vi "configuration UI.vi"() -> ()   [LabVIEW 2013, in "Modbus Slave editor node.lvclass"]
doc: "Platypus Framework 1.0.1.65\nNI Systems Engineering - National Instruments"
uses:
  Modbus Slave editor node.lvclass
  <vilib>/NI/Configuration Framework/Node/NodeRef.ctl
  <vilib>/NI/Configuration Framework/Node/NISE_CEF_Node.lvclass
  <vilib>/NI/AMC/Message Queue.ctl
  <vilib>/NI/AMC/Message.ctl
  <vilib>/NI/Tools/Keyed Array/KeyedArray.ctl
  <vilib>/NI/Configuration Framework/Node/UserEventRef.ctl
  <vilib>/NI/Configuration Framework/Controls/EventCluster.ctl
  module/configuration/modbus mapping behavior.ctl
  module/configuration/modbus class.ctl
  <vilib>/NI/Module Execution Interface/Engine Configuration/engine configuration.lvclass
  module/configuration/Modbus Slave configuration.lvclass
  <vilib>/NI/Tag Bus Data Framework/Configuration Editor/Classes/Engine Parent/Engine Parent Editor Node.lvclass
  <vilib>/NI/Tag Bus/tag/tag descriptor.lvclass
  <vilib>/NI/Tag Bus/tag/Data Type.ctl
  <vilib>/NI/Tag Bus/tag/tag descriptor.lvclass/tag descriptor.ctl
  <vilib>/NI/Configuration Framework/serializable configuration/NISE_CEF_serializable configuration.lvclass/NISE_CEF_serializable configuration.ctl
  <vilib>/NI/Configuration Framework/serializable configuration/NISE_CEF_serializable configuration.lvclass
  module/configuration/Modbus Slave configuration.lvclass/Modbus Slave configuration.ctl
  Modbus Slave editor node.lvclass/Modbus Slave editor node.ctl
  <vilib>/NI/Tag Bus/tag/write data type.vi
  module/configuration/Write port (502).vi
  module/configuration/Write baud rate.vi
  module/configuration/Write class.vi
  module/configuration/Write flow control (none).vi
  module/configuration/Write parity (even).vi
  module/configuration/Write serial type.vi
  module/configuration/Write unit ID.vi
  module/configuration/Write VISA resource name.vi
  module/configuration/Write IP address.vi
  module/configuration/Read modbus channels.vi
  module/configuration/Read port (502).vi
  module/configuration/Read baud rate.vi
  module/configuration/Read class.vi
  module/configuration/Read flow control (none).vi
  module/configuration/Read parity (even).vi
  module/configuration/Read serial type.vi
  module/configuration/Read unit ID.vi
  module/configuration/Read VISA resource name.vi
  module/configuration/Read IP address.vi
  <vilib>/NI/Tag Bus Data Framework/Configuration Editor/Classes/Module editor node/Read Module Configuration.vi
  <vilib>/NI/Tag Bus Module Framework/module configuration/TBM module configuration.lvclass
  module/module channel/Modbus Module Channel.lvclass
  <vilib>/NI/Configuration Framework/NISE_CEF_TreeControl.lvlib
  <vilib>/NI/Tag Bus Data Framework/Configuration Editor/Classes/Module editor node/module editor node.lvclass
  <vilib>/NI/Tools/Keyed Array/Tools_KeyedArray.lvlib
  <vilib>/NI/AMC/AMC.lvlib
panel:
  in  "export":bool
  in  "Tab Control":T1(tab)
  in  "hidden_remove":bool
  in  "hidden_settings":bool
  in  "hidden_Add":bool
  in  "Remove Button":bool
  in  "Add Button":bool
  in  "channel":i32(listbox)=1
  in  "settings":bool
  in  "address":string
  in  "port (502)":u16=502
  in  "baud rate":u32
  in  "class":T2
  in  "flow control (none)":u16
  in  "parity (even)":u16
  in  "serial type":enum16{"RTU", "ASCII"}(ring)
  in  "unit ID":u8
  in  "VISA resource name":refnum<visa-resource-name>
  in  "remap":bool
  in  "mapping":T3
  in  "user event":T4
  in  "main queue":T5
  in  "node ref":T6
  # "TCP"
  # "TCP Master"
  # "Serial"
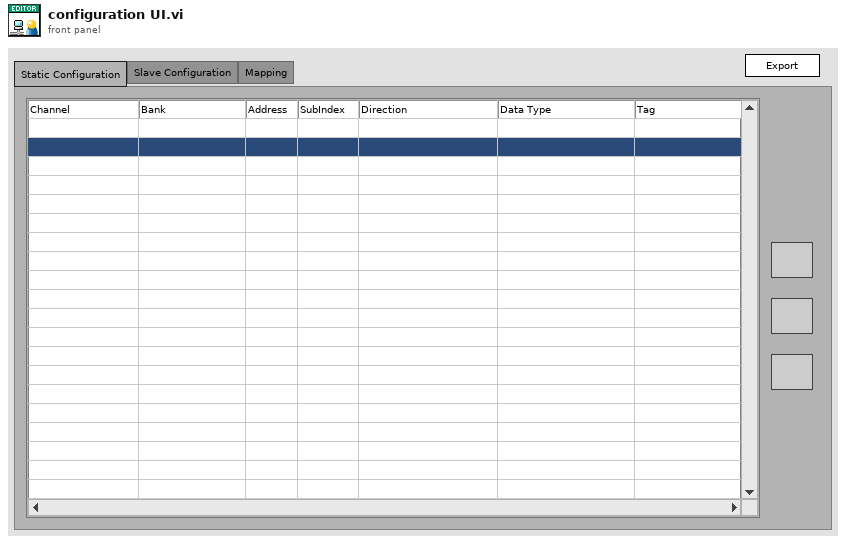
[diagram p1: front panel]
types:
  T1 = enum32{"Static Configuration", "Slave Configuration", "Mapping"}
  T2 = typedef "Modbus Slave configuration.lvclass/modbus class.ctl" = enum16{"TCP master", "TCP slave", "serial master", "serial slave"}
  T3 = typedef "Modbus Slave configuration.lvclass/modbus mapping behavior.ctl" = enum16{"custom", "optimized"}
  T4 = typedef "NISE_CEF_Node.lvclass/UserEventRef.ctl" = refnum<user-event>
  T5 = typedef "AMC.lvlib/Message Queue.ctl" = refnum<queue>
  T6 = typedef "NISE_CEF_Node.lvclass/NodeRef.ctl" = refnum<data-value>
  T7 = typedef "NISE_CEF_TreeControl.lvlib/EventCluster.ctl" = cluster{"command":string, "data":string}
  T8 = typedef "tag bus.lvlib/tag descriptor.lvclass/Data Type.ctl" = enum16{"Double", "Single", "I64", "I32", "I16", "I8", "U64", "U32", "U16", "U8", "Boolean", "String", "Array of Double", "Array of Single", "Array of I64", "Array of I32", "Array of I16", "Array of I8", "Array of U64", "Array of U32", "Array of U16", "Array of U8", "Array of Boolean", "Array of String"}
  T9 = typedef "Modbus Slave editor node.lvclass/table line.ctl" = cluster{"mbchan":refnum<class "Modbus Module Channel.lvclass">, "tag name":string}
  T10 = typedef "LVPoint32TypeDef.ctl" = cluster{"Horizontal":i32, "Vertical":i32}
  T11 = typedef "LVRowAndColumnTypeDef.ctl" = cluster{"Row":i32, "Column":i32}
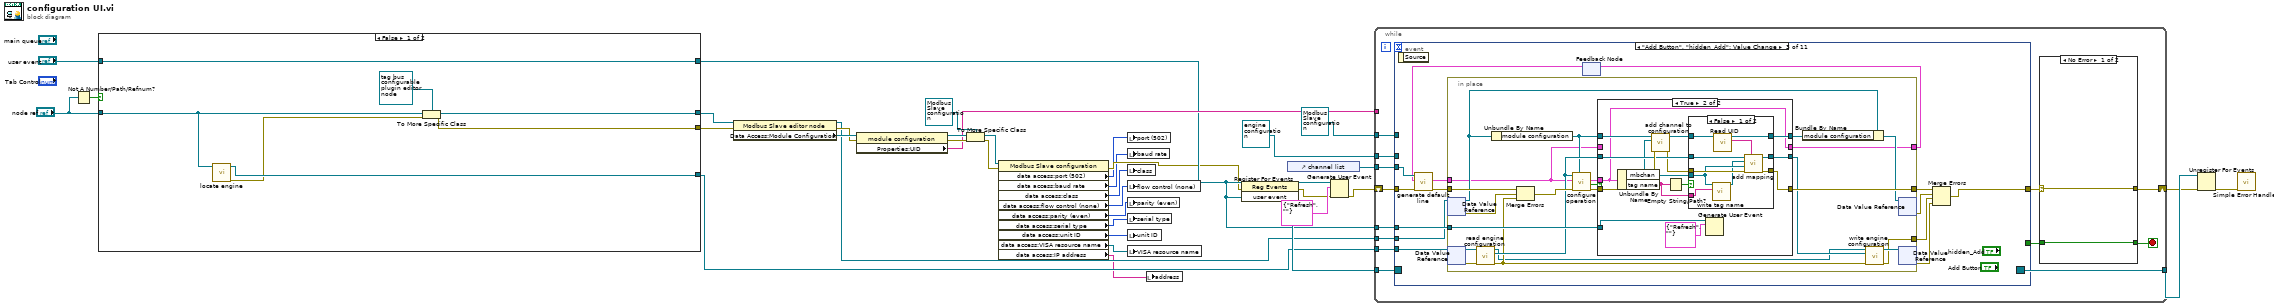
[diagram p0: block diagram]
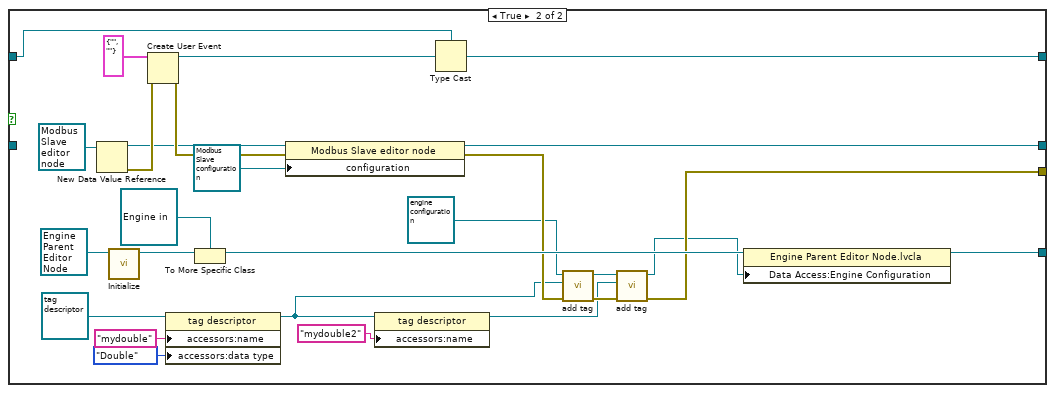
[diagram p2: hidden frame]
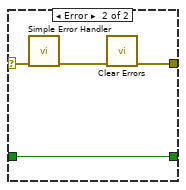
[diagram p3: hidden frame]
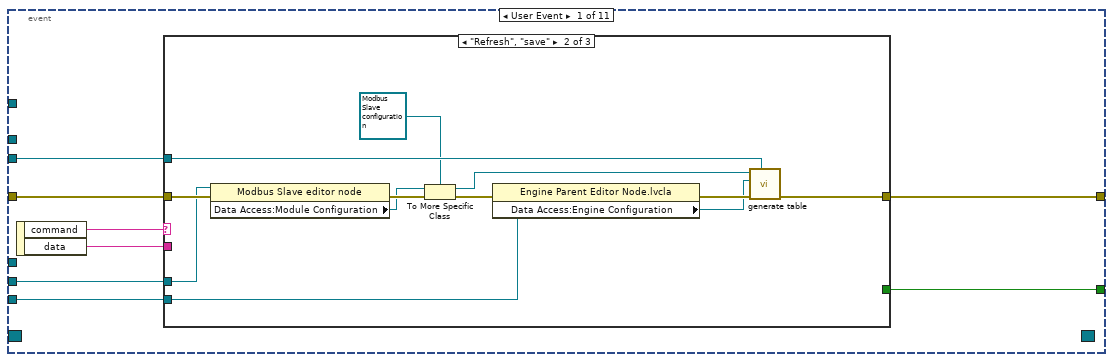
[diagram p4: hidden frame]
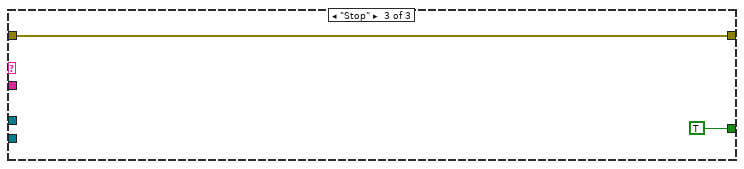
[diagram p6: hidden frame]
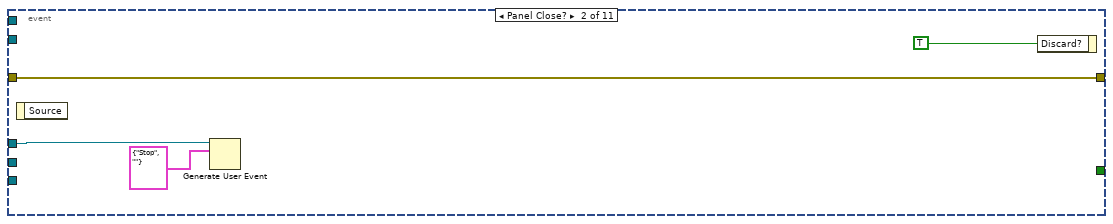
[diagram p7: hidden frame]
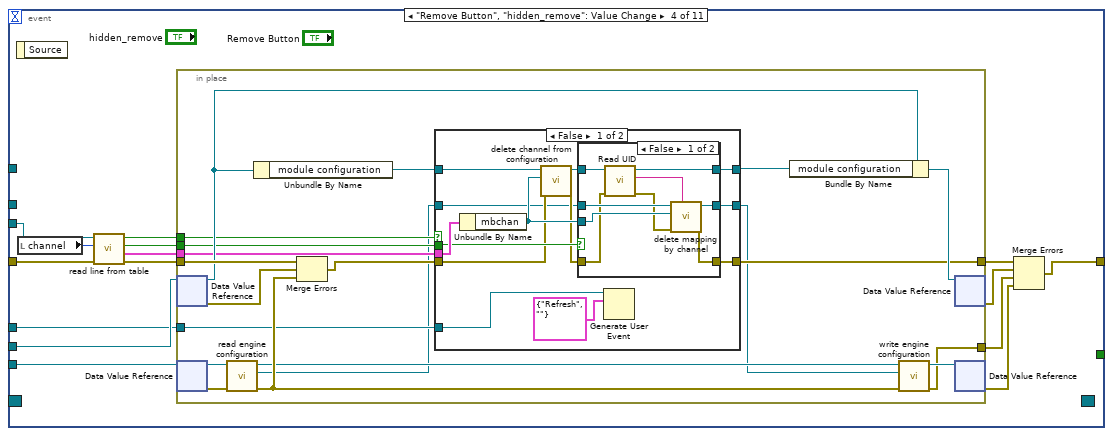
[diagram p10: hidden frame]
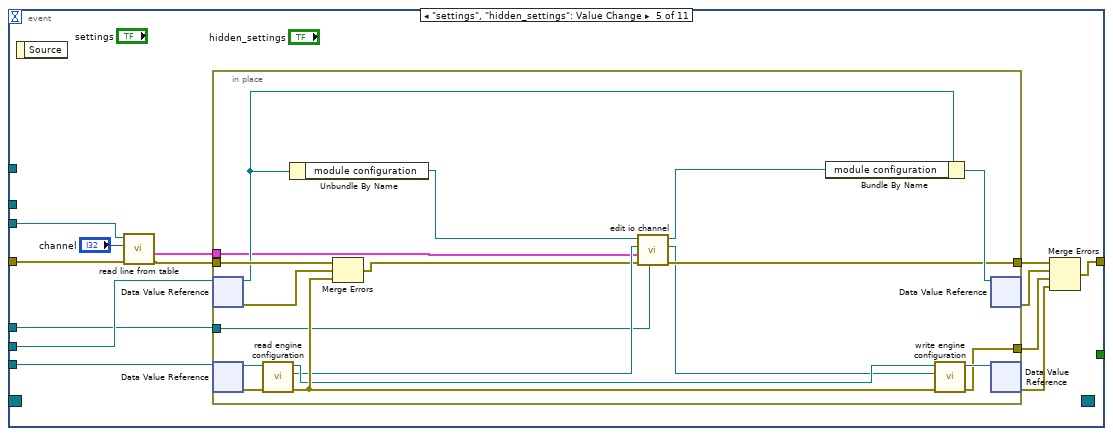
[diagram p13: hidden frame]
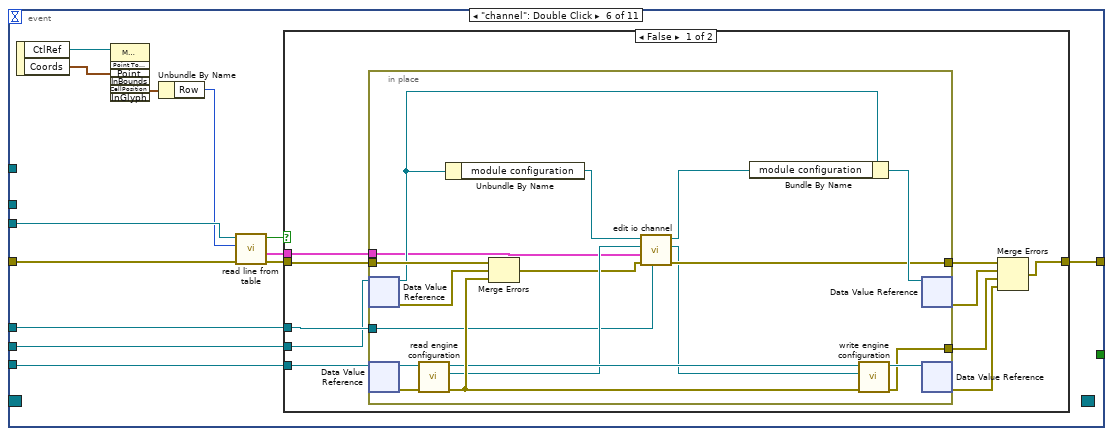
[diagram p14: hidden frame]
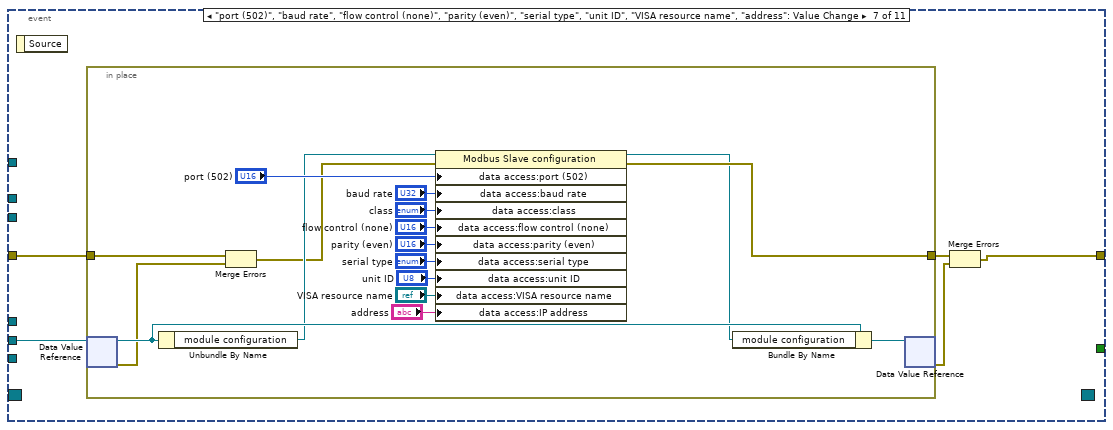
[diagram p16: hidden frame]
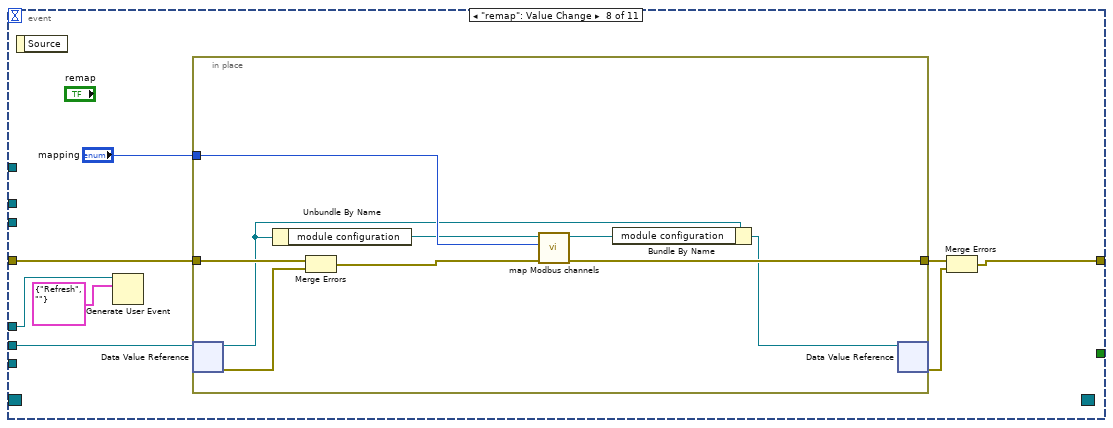
[diagram p17: hidden frame]
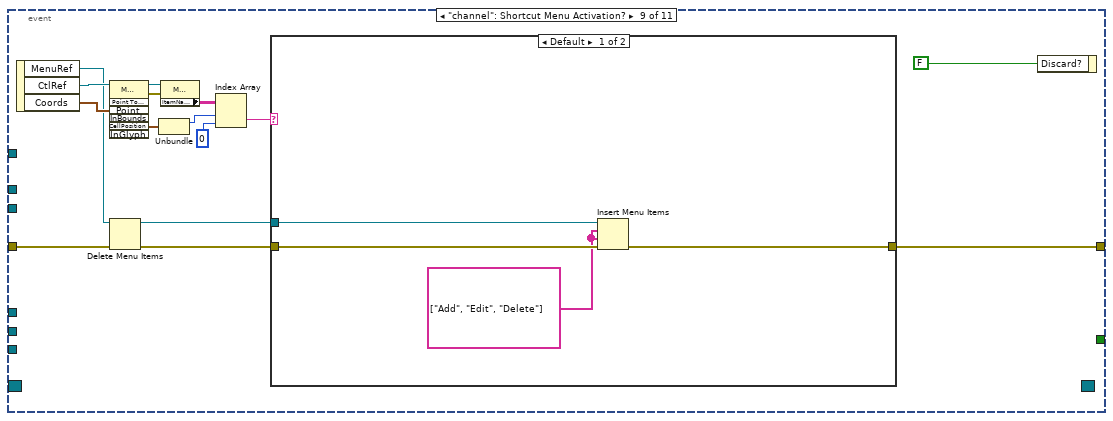
[diagram p18: hidden frame]
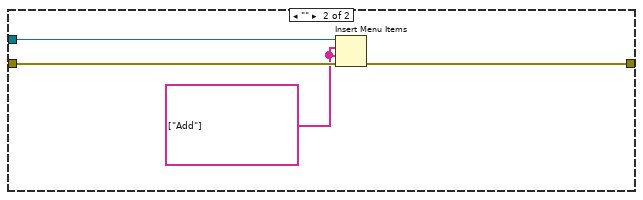
[diagram p19: hidden frame]
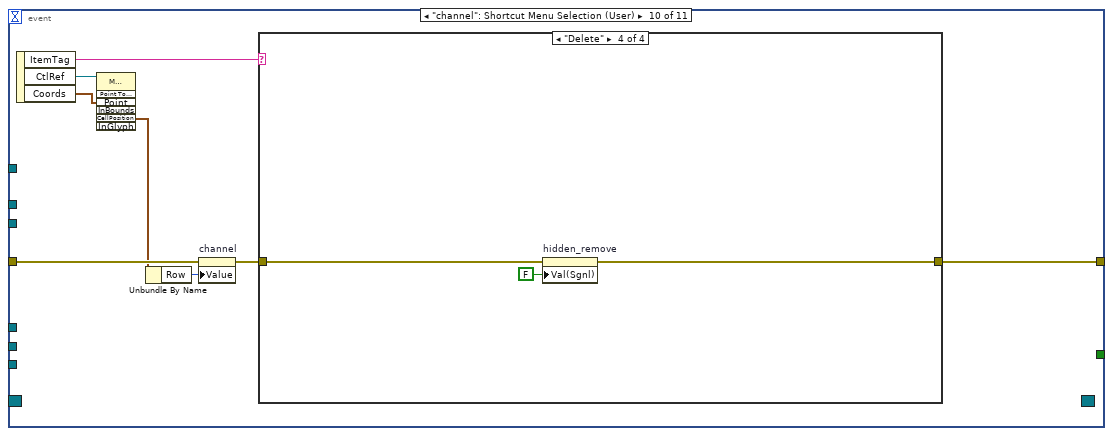
[diagram p20: hidden frame]
diagram:
  n1 = Not A Number/Path/Refnum?(number/path/refnum="node ref") -> (NaN/Path/Refnum?=w28:bool)
  n2 = case shown="False" w28 {
    tunnel: "user event" -> [w43 w47]
    tunnel: [w43 w48] -> w15
    tunnel: "node ref" -> [w41 _]
    tunnel: [w40 w64] -> w23
    tunnel: [w39 w51] -> w26
    tunnel: [w38 w45] -> w21
    frame False {
      n3 = call <vilib>:"locate engine.vi"("component"=w41) -> ("error out"=w37:errorcluster, "engine"=w38:refnum<data-value>)  [unwired: 9 in]
      n4 = To More Specific Class(target class=refnum<data-value> refnum ("data value reference"), reference=w41, error in=w37) -> (specific class reference=w40:refnum<data-value>, error out=w39:errorcluster)
    }
    frame True {
      n5 = New Data Value Reference(data value=refnum<class "Modbus Slave editor node.lvclass"> refnum ("tag bus configurable plugin editor node")) -> (data value reference=w63:refnum<data-value>, error out=w66:errorcluster)  [unwired: 1 in]
      n6 = call-dynamic "Initialize.vi"("Engine in"=refnum<class "Engine Parent Editor Node.lvclass"> refnum) -> ("data value reference"=w62:T6)  [unwired: 8 in, 2 out]
      n7 = Create User Event(user event datatype=T7 {"command"="", "data"=""} ("event data"), error in=w66) -> (user event=w69:refnum<user-event>, error out=w65:errorcluster)
      n8 = property class="tag descriptor"(reference=refnum<class "tag descriptor.lvclass"> refnum ("tag descriptor"), "accessors:name"="mydouble" ("name"), "accessors:data type"=Data_Type."Double" ("data type")) -> (reference out=w49:refnum<class "tag descriptor.lvclass">)  [unwired: 1 in, 1 out]
      n9 = To More Specific Class(target class=refnum<data-value> refnum ("data value reference"), reference=w62) -> (specific class reference=w61:refnum<data-value>)  [unwired: 1 in, 1 out]
      n10 = property class="Modbus Slave editor node"(reference=w63, error in=w65, "configuration"=refnum<class "Modbus Slave configuration.lvclass"> refnum ("tag bus configurable plugin module configuration")) -> (reference out=w64:refnum<data-value>, error out=w55:errorcluster)
      n11 = property class="tag descriptor"(reference=w49, "accessors:name"="mydouble2" ("name")) -> (reference out=w50:refnum<class "tag descriptor.lvclass">)  [unwired: 1 in, 1 out]
      n12 = Type Cast(type=w47, x=w69) -> (*(type *) &x=w48:T4)
      n13 = call <vilib>:"add tag.vi"("error in"=w55, "tag descriptor"=w49, "engine configuration in"=refnum<class "engine configuration.lvclass"> refnum ("Engine Configuration")) -> ("error out"=w53:errorcluster, "engine configuration out"=w52:refnum<class "engine configuration.lvclass">)  [unwired: 7 in]
      n14 = call <vilib>:"add tag.vi"("error in"=w53, "tag descriptor"=w50, "engine configuration in"=w52) -> ("error out"=w51:errorcluster, "engine configuration out"=w44:refnum<class "engine configuration.lvclass">)  [unwired: 7 in]
      n15 = property class="Engine Parent Editor Node.lvcla"(reference=w61, "Data Access:Engine Configuration"=w44) -> (reference out=w45:refnum<data-value>)  [unwired: 1 in, 1 out]
    }
  }
  n16 = property class="Modbus Slave editor node"(reference=w23, error in=w26) -> (reference out=w22:refnum<data-value>, error out=w31:errorcluster, "Data Access:Module Configuration"=w32:refnum<class "TBM module configuration.lvclass">)
  n17 = property class="module configuration"(reference=w32, error in=w31) -> (reference out=w29:refnum<class "TBM module configuration.lvclass">, error out=w30:errorcluster, "Properties:UID"=w25:string)
  n18 = To More Specific Class(target class=refnum<class "Modbus Slave configuration.lvclass"> refnum ("tag bus configurable plugin module configuration"), reference=w29, error in=w30) -> (specific class reference=w12:refnum<class "Modbus Slave configuration.lvclass">, error out=w11:errorcluster)
  n19 = property class="Modbus Slave configuration"(reference=w12, error in=w11) -> (error out=w10:errorcluster, "data access:port (502)"=w5:u16, "data access:baud rate"=w9:u32, "data access:class"=w6:T2, "data access:flow control (none)"=w4:u16, "data access:parity (even)"=w3:u16, "data access:serial type"=w2:enum16{"RTU", "ASCII"}, "data access:unit ID"=w7:u8, "data access:VISA resource name"=w8:refnum<visa-resource-name>, "data access:IP address"=w1:string)  [unwired: 1 out]
  n20 = local write "port (502)"(w5) -> ()
  n21 = local write "baud rate"(w9) -> ()
  n22 = local write "class"(w6) -> ()
  n23 = local write "flow control (none)"(w4) -> ()
  n24 = local write "parity (even)"(w3) -> ()
  n25 = local write "serial type"(w2) -> ()
  n26 = local write "unit ID"(w7) -> ()
  n27 = local write "VISA resource name"(w8) -> ()
  n28 = local write "address"(w1) -> ()
  n29 = register-events(error in=w10, w15) -> (reference out=w36:refnum<event-registration>, error out=w14:errorcluster)  [unwired: 1 in]
  n30 = control-ref of="channel list"() -> (w19:refnum<vi>)
  n31 = Generate User Event(user event=w15, event data cluster=T7 {"command"="Refresh", "data"=""} ("event data"), error in=w14) -> (error out=w13:errorcluster)  [unwired: 1 in, 1 out]
  n32 = while {
    tunnel: w36 -> [w83]
    tunnel: [w82] -> w35
    shift-right: [w79] -> w34
    shift-left: w13 -> [w81]
    tunnel: w25 -> [_]
    tunnel: w22 -> [w76]
    tunnel: w21 -> [w75]
    tunnel: w15 -> [w74]
    tunnel: w19 -> [w72]
    tunnel: refnum<class "Modbus Slave configuration.lvclass"> refnum ("tag bus configurable plugin module configuration") -> [w78]
    tunnel: refnum<class "engine configuration.lvclass"> refnum ("Engine Configuration") -> [w77]
    stop <- w80 stop-if-true
    n33 = event shown="[2] \"Add Button\", \"hidden_Add\": Value Change" {
      selector: w83 -> [_ _ _ _ _ _ _ _ _ _ _]
      dyn-events: [_ _ _ _ _ _ _ _ _ _ _] -> w82
      timeout: _ -> [_ _ _ _ _ _ _ _ _ _ _]
      tunnel: [w97 _ _ _ _ _ _ _ _ _ _] -> w71
      tunnel: [w91 w116 w124 w187 w252 w289 w321 w344 w359 w386 w408] -> w73
      tunnel: w81 -> [w92 w116 w129 w198 w259 w290 w324 w349 w373 w385 w413]
      tunnel: w78 -> [_ _ _ _ _ _ _ _ _ _ _]
      tunnel: w77 -> [_ _ _ _ _ _ _ _ _ _ _]
      tunnel: w76 -> [w95 _ w120 w189 w248 w279 w322 w342 _ _ w406]
      tunnel: w75 -> [w94 _ w123 w190 w249 w278 _ _ _ _ _]
      tunnel: w74 -> [_ w113 w126 w188 w247 w286 _ w347 _ _ _]
      tunnel: w72 -> [w90 _ w125 w196 w257 w285 _ _ _ _ _]
      event User Event {
        n34 = event-data() -> ("command"=w96:string, "data"=w93:string)  [unwired: 1 in]
        n35 = case shown="\"Refresh\", \"save\"" w96 {
          tunnel: [_ _ TRUE] -> w97
          tunnel: w95 -> [_ w105 _]
          tunnel: w94 -> [_ w104 _]
          tunnel: w93 -> [_ _ _]
          tunnel: w92 -> [w98 w110 w111]
          tunnel: [w98 w109 w111] -> w91
          tunnel: w90 -> [_ w108 _]
          frame Default {
          }
          frame "Refresh", "save" {
            n36 = property class="Modbus Slave editor node"(reference=w105, error in=w110) -> (error out=w106:errorcluster, "Data Access:Module Configuration"=w100:refnum<class "TBM module configuration.lvclass">)  [unwired: 1 out]
            n37 = To More Specific Class(target class=refnum<class "Modbus Slave configuration.lvclass"> refnum ("tag bus configurable plugin module configuration"), reference=w100, error in=w106) -> (specific class reference=w99:refnum<class "Modbus Slave configuration.lvclass">, error out=w102:errorcluster)
            n38 = property class="Engine Parent Editor Node.lvcla"(reference=w104, error in=w102) -> (error out=w107:errorcluster, "Data Access:Engine Configuration"=w103:refnum<class "engine configuration.lvclass">)  [unwired: 1 out]
            n39 = call "generate table.vi"("table"=w108, "error in"=w107, "engine configuration"=w103, "tag bus configurable plugin module configuration"=w99) -> ("error out"=w109:errorcluster)  [unwired: 7 in]
          }
          frame "Stop" {
          }
        }
      }
      event Panel Close? {
        n40 = event-data() -> ()  [unwired: 1 in, 1 out]
        n41 = Generate User Event(user event=w113, event data cluster=T7 {"command"="Stop", "data"=""} ("event data")) -> ()  [unwired: 2 in, 2 out]
        n42 = event-data("Discard?"=TRUE) -> ()  [unwired: 1 in, 1 out]
      }
      event "Add Button", "hidden_Add": Value Change {
        n43 = event-data() -> ()  [unwired: 1 in, 1 out]
        n44 = feedback #1() -> (w117:T9)  [unwired: 1 in]
        n45 = call "generate default line.vi"("error in"=w129, "last line"=w117, "operations table"=w125) -> ("error out"=w127:errorcluster, "line"=w128:T9)  [unwired: 7 in]
        n46 = in-place {
          in-place-border: [w152] -> w130
          in-place-border: w128 -> [w132]
          in-place-border: w127 -> [w151]
          in-place-border: w126 -> [w147]
          in-place-border: [w138] -> w121
          in-place-border: [w131] -> w118
          n47 = in-place-dvr #2(w120) -> (w133:refnum<class "Modbus Slave editor node.lvclass">, w137:errorcluster)
          n48 = in-place-dvr #3(w123) -> (w145:refnum<class "Engine Parent Editor Node.lvclass">, w144:errorcluster)
          n49 = call <vilib>:"read engine configuration.vi"("error in"=w144, "Engine Parent Editor Node in"=w145) -> ("error out"=w140:errorcluster, "engine configuration"=w143:refnum<class "engine configuration.lvclass">, "Engine Parent Editor Node out"=w139:refnum<class "Engine Parent Editor Node.lvclass">)  [unwired: 7 in]
          n50 = Unbundle By Name(w133) -> ("module configuration"=w136:refnum<class "Modbus Slave configuration.lvclass">)
          n51 = Merge Errors(w151, w137, w140) -> (w146:errorcluster)
          n52 = call "configure operation.vi"("tag bus configurable plugin module configuration"=w136, "error in"=w146, "line item in"=w132, "engine configuration"=w143) -> ("error out"=w149:errorcluster, "success"=w148:bool, "line item out"=w150:T9)  [unwired: 4 in, 1 out]
          n53 = case shown="True" w148 {
            tunnel: [w156 w160] -> w152
            tunnel: w149 -> [w156 w169]
            tunnel: w143 -> [w155 w167]
            tunnel: w150 -> [_ w157]
            tunnel: w136 -> [w154 w170]
            tunnel: [w155 w166] -> w141
            tunnel: [w154 w161] -> w135
            tunnel: w147 -> [_ w159]
            tunnel: w132 -> [w153 _]
            tunnel: [w153 w157] -> w131
            frame False {
            }
            frame True {
              n54 = Unbundle By Name(w157) -> ("mbchan"=w164:refnum<class "Modbus Module Channel.lvclass">, "tag name"=w163:string)
              n55 = call "add channel to configuration.vi"("error in"=w169, "Modbus Module Channel.lvclass"=w164, "Modbus Slave configuration in"=w170) -> ("error out"=w165:errorcluster, "Modbus Slave configuration out"=w162:refnum<class "Modbus Slave configuration.lvclass">)  [unwired: 7 in]
              n56 = Empty String/Path?(string/path=w163) -> (empty?=w168:bool)
              n57 = case shown="False" w168 {
                tunnel: w167 -> [w180 w183]
                tunnel: [w179 w183] -> w166
                tunnel: w165 -> [w178 w182]
                tunnel: w164 -> [w175 _]
                tunnel: w163 -> [w173 _]
                tunnel: [w177 w182] -> w160
                tunnel: w162 -> [w176 w181]
                tunnel: [w172 w181] -> w161
                frame False {
                  n58 = call <vilib>:"write tag name.vi"("name"=w173, "system tag in"=w175) -> ("system tag out"=w174:refnum<class "Modbus Module Channel.lvclass">)  [unwired: 8 in, 1 out]
                  n59 = call <vilib>:"Read UID.vi"("configuration in"=w176) -> ("instance id"=w171:string, "configuration out"=w172:refnum<class "Modbus Slave configuration.lvclass">)  [unwired: 8 in, 1 out]
                  n60 = call <vilib>:"add mapping.vi"("owner ID"=w171, "error in"=w178, "channel"=w175, "tag descriptor"=w174, "engine configuration"=w180) -> ("error out"=w177:errorcluster, "engine configuration out"=w179:refnum<class "engine configuration.lvclass">)  [unwired: 5 in]
                }
                frame True {
                }
              }
              n61 = Generate User Event(user event=w159, event data cluster=T7 {"command"="Refresh", "data"=""} ("event data")) -> ()  [unwired: 2 in, 2 out]
            }
          }
          n62 = Bundle By Name(cluster=w133, "module configuration"=w135) -> (w134:refnum<class "Modbus Slave editor node.lvclass">)
          n63 = call <vilib>:"write engine configuration.vi"("error in"=w140, "engine configuration"=w141, "Engine Parent Editor Node in"=w139) -> ("error out"=w138:errorcluster, "Engine Parent Editor Node out"=w142:refnum<class "Engine Parent Editor Node.lvclass">)  [unwired: 7 in]
          n64 = in-place-dvr #2(w134) -> (w119:errorcluster)  [unwired: 1 out]
          n65 = in-place-dvr #3(w142) -> (w122:errorcluster)  [unwired: 1 out]
        }
        n66 = feedback-in #1(w118) -> ()
        n67 = Merge Errors(w130, w119, w121, w122) -> (w124:errorcluster)
      }
      event "Remove Button", "hidden_remove": Value Change {
        n68 = event-data() -> ()  [unwired: 1 in, 1 out]
        n69 = local read "channel"() -> (w197:i32)
        n70 = call "read line from table.vi"("error in"=w198, "line number"=w197, "channels table"=w196) -> ("error out"=w192:errorcluster, "line"=w191:T9, "empty tag?"=w185:bool, "empty channel?"=w184:bool)  [unwired: 5 in]
        n71 = in-place {
          in-place-border: w191 -> [w203]
          in-place-border: w192 -> [w218]
          in-place-border: w188 -> [w206]
          in-place-border: [w212] -> w194
          in-place-border: [w207] -> w186
          in-place-border: w185 -> [w202]
          in-place-border: w184 -> [w201]
          n72 = in-place-dvr #4(w189) -> (w209:refnum<class "Modbus Slave editor node.lvclass">, w211:errorcluster)
          n73 = in-place-dvr #5(w190) -> (w217:refnum<class "Engine Parent Editor Node.lvclass">, w216:errorcluster)
          n74 = call <vilib>:"read engine configuration.vi"("error in"=w216, "Engine Parent Editor Node in"=w217) -> ("error out"=w214:errorcluster, "engine configuration"=w200:refnum<class "engine configuration.lvclass">, "Engine Parent Editor Node out"=w213:refnum<class "Engine Parent Editor Node.lvclass">)  [unwired: 7 in]
          n75 = Unbundle By Name(w209) -> ("module configuration"=w205:refnum<class "Modbus Slave configuration.lvclass">)
          n76 = Merge Errors(w218, w211, w214) -> (w208:errorcluster)
          n77 = case shown="False" w201 {
            tunnel: [w221 w245] -> w207
            tunnel: w203 -> [w231 _]
            tunnel: w205 -> [w229 w244]
            tunnel: w200 -> [w224 w246]
            tunnel: w202 -> [w230 _]
            tunnel: w208 -> [w227 w245]
            tunnel: [w223 w246] -> w199
            tunnel: [w222 w244] -> w204
            tunnel: w206 -> [w219 _]
            frame False {
              n78 = Unbundle By Name(w231) -> ("mbchan"=w228:refnum<class "Modbus Module Channel.lvclass">)
              n79 = call "delete channel from configuration.vi"("error in"=w227, "Modbus Module Channel.lvclass"=w228, "Modbus Slave configuration in"=w229) -> ("error out"=w225:errorcluster, "Modbus Slave configuration out"=w226:refnum<class "Modbus Slave configuration.lvclass">)  [unwired: 7 in]
              n80 = case shown="False" w230 {
                tunnel: w228 -> [w239 _]
                tunnel: w226 -> [w234 w241]
                tunnel: w225 -> [w238 w242]
                tunnel: w224 -> [w240 w243]
                tunnel: [w237 w243] -> w223
                tunnel: [w236 w242] -> w221
                tunnel: [w233 w241] -> w222
                frame False {
                  n81 = call <vilib>:"Read UID.vi"("error in"=w238, "configuration in"=w234) -> ("error out"=w235:errorcluster, "instance id"=w232:string, "configuration out"=w233:refnum<class "Modbus Slave configuration.lvclass">)  [unwired: 7 in]
                  n82 = call <vilib>:"delete mapping by channel.vi"("owner ID"=w232, "error in"=w235, "channel"=w239, "engine configuration in"=w240) -> ("error out"=w236:errorcluster, "engine configuration out"=w237:refnum<class "engine configuration.lvclass">)  [unwired: 6 in]
                }
                frame True {
                }
              }
              n83 = Generate User Event(user event=w219, event data cluster=T7 {"command"="Refresh", "data"=""} ("event data")) -> ()  [unwired: 2 in, 2 out]
            }
            frame True {
            }
          }
          n84 = Bundle By Name(cluster=w209, "module configuration"=w204) -> (w210:refnum<class "Modbus Slave editor node.lvclass">)
          n85 = call <vilib>:"write engine configuration.vi"("error in"=w214, "engine configuration"=w199, "Engine Parent Editor Node in"=w213) -> ("error out"=w212:errorcluster, "Engine Parent Editor Node out"=w215:refnum<class "Engine Parent Editor Node.lvclass">)  [unwired: 7 in]
          n86 = in-place-dvr #4(w210) -> (w193:errorcluster)  [unwired: 1 out]
          n87 = in-place-dvr #5(w215) -> (w195:errorcluster)  [unwired: 1 out]
        }
        n88 = Merge Errors(w186, w193, w194, w195) -> (w187:errorcluster)
      }
      event "settings", "hidden_settings": Value Change {
        n89 = event-data() -> ()  [unwired: 1 in, 1 out]
        n90 = call "read line from table.vi"("error in"=w259, "line number"="channel", "channels table"=w257) -> ("error out"=w251:errorcluster, "line"=w250:T9)  [unwired: 5 in, 2 out]
        n91 = in-place {
          in-place-border: [w267] -> w256
          in-place-border: w250 -> [w260]
          in-place-border: w251 -> [w277]
          in-place-border: w247 -> [w262]
          in-place-border: [w271] -> w254
          n92 = in-place-dvr #6(w248) -> (w268:refnum<class "Modbus Slave editor node.lvclass">, w270:errorcluster)
          n93 = in-place-dvr #7(w249) -> (w276:refnum<class "Engine Parent Editor Node.lvclass">, w275:errorcluster)
          n94 = call <vilib>:"read engine configuration.vi"("error in"=w275, "Engine Parent Editor Node in"=w276) -> ("error out"=w273:errorcluster, "engine configuration"=w263:refnum<class "engine configuration.lvclass">, "Engine Parent Editor Node out"=w272:refnum<class "Engine Parent Editor Node.lvclass">)  [unwired: 7 in]
          n95 = Unbundle By Name(w268) -> ("module configuration"=w265:refnum<class "Modbus Slave configuration.lvclass">)
          n96 = Merge Errors(w277, w270, w273) -> (w261:errorcluster)
          n97 = call "edit io channel.vi"("user event"=w262, "error in"=w261, "line"=w260, "engine configuration in"=w263, "tag bus configurable plugin module configuration in"=w265) -> ("error out"=w267:errorcluster, "engine configuration"=w264:refnum<class "engine configuration.lvclass">, "tag bus configurable plugin module configuration out"=w266:refnum<class "Modbus Slave configuration.lvclass">)  [unwired: 4 in]
          n98 = Bundle By Name(cluster=w268, "module configuration"=w266) -> (w269:refnum<class "Modbus Slave editor node.lvclass">)
          n99 = call <vilib>:"write engine configuration.vi"("error in"=w273, "engine configuration"=w264, "Engine Parent Editor Node in"=w272) -> ("error out"=w271:errorcluster, "Engine Parent Editor Node out"=w274:refnum<class "Engine Parent Editor Node.lvclass">)  [unwired: 7 in]
          n100 = in-place-dvr #6(w269) -> (w253:errorcluster)  [unwired: 1 out]
          n101 = in-place-dvr #7(w274) -> (w255:errorcluster)  [unwired: 1 out]
        }
        n102 = Merge Errors(w256, w253, w254, w255) -> (w252:errorcluster)
      }
      event "channel": Double Click {
        n103 = event-data() -> ("CtlRef"=w284:refnum<vi>, "Coords"=w283:T10)  [unwired: 1 in]
        n104 = invoke class="MCListbox (strict)" method="Point To Row Column"(reference=w284, "Point"=w283) -> ("CellPosition"=w282:T11)  [unwired: 5 in, 6 out]
        n105 = Unbundle By Name(w282) -> ("Row"=w281:i32)
        n106 = call "read line from table.vi"("error in"=w290, "line number"=w281, "channels table"=w285) -> ("error out"=w288:errorcluster, "line"=w287:T9, "empty channel?"=w280:bool)  [unwired: 5 in, 1 out]
        n107 = case shown="False" w280 {
          tunnel: [w295 w319] -> w289
          tunnel: w288 -> [w296 w319]
          tunnel: w287 -> [w293 _]
          tunnel: w286 -> [w294 _]
          tunnel: w279 -> [w292 _]
          tunnel: w278 -> [w291 _]
          frame False {
            n108 = in-place {
              in-place-border: [w306] -> w297
              in-place-border: w296 -> [w318]
              in-place-border: w294 -> [w303]
              in-place-border: [w312] -> w299
              in-place-border: w293 -> [w301]
              n109 = in-place-dvr #8(w292) -> (w309:refnum<class "Modbus Slave editor node.lvclass">, w311:errorcluster)
              n110 = in-place-dvr #9(w291) -> (w317:refnum<class "Engine Parent Editor Node.lvclass">, w316:errorcluster)
              n111 = call <vilib>:"read engine configuration.vi"("error in"=w316, "Engine Parent Editor Node in"=w317) -> ("error out"=w314:errorcluster, "engine configuration"=w305:refnum<class "engine configuration.lvclass">, "Engine Parent Editor Node out"=w313:refnum<class "Engine Parent Editor Node.lvclass">)  [unwired: 7 in]
              n112 = Unbundle By Name(w309) -> ("module configuration"=w308:refnum<class "Modbus Slave configuration.lvclass">)
              n113 = Merge Errors(w318, w311, w314) -> (w302:errorcluster)
              n114 = call "edit io channel.vi"("user event"=w303, "error in"=w302, "line"=w301, "engine configuration in"=w305, "tag bus configurable plugin module configuration in"=w308) -> ("error out"=w306:errorcluster, "engine configuration"=w304:refnum<class "engine configuration.lvclass">, "tag bus configurable plugin module configuration out"=w307:refnum<class "Modbus Slave configuration.lvclass">)  [unwired: 4 in]
              n115 = Bundle By Name(cluster=w309, "module configuration"=w307) -> (w310:refnum<class "Modbus Slave editor node.lvclass">)
              n116 = call <vilib>:"write engine configuration.vi"("error in"=w314, "engine configuration"=w304, "Engine Parent Editor Node in"=w313) -> ("error out"=w312:errorcluster, "Engine Parent Editor Node out"=w315:refnum<class "Engine Parent Editor Node.lvclass">)  [unwired: 7 in]
              n117 = in-place-dvr #8(w310) -> (w300:errorcluster)  [unwired: 1 out]
              n118 = in-place-dvr #9(w315) -> (w298:errorcluster)  [unwired: 1 out]
            }
            n119 = Merge Errors(w297, w300, w299, w298) -> (w295:errorcluster)
          }
          frame True {
          }
        }
      }
      event "port (502)", "baud rate", "flow control (none)", "parity (even)", "serial type", "unit ID", "VISA resource name", "address": Value Change {
        n120 = event-data() -> ()  [unwired: 1 in, 1 out]
        n121 = in-place {
          in-place-border: w324 -> [w341]
          in-place-border: [w340] -> w323
          n122 = in-place-dvr #10(w322) -> (w338:refnum<class "Modbus Slave editor node.lvclass">, w333:errorcluster)
          n123 = Unbundle By Name(w338) -> ("module configuration"=w336:refnum<class "Modbus Slave configuration.lvclass">)
          n124 = Merge Errors(w341, w333) -> (w334:errorcluster)
          n125 = property class="Modbus Slave configuration"(reference=w336, error in=w334, "data access:port (502)"="port (502)", "data access:baud rate"="baud rate", "data access:class"="class", "data access:flow control (none)"="flow control (none)", "data access:parity (even)"="parity (even)", "data access:serial type"="serial type", "data access:unit ID"="unit ID", "data access:VISA resource name"="VISA resource name", "data access:IP address"="address") -> (reference out=w335:refnum<class "Modbus Slave configuration.lvclass">, error out=w340:errorcluster)
          n126 = Bundle By Name(cluster=w338, "module configuration"=w335) -> (w337:refnum<class "Modbus Slave editor node.lvclass">)
          n127 = in-place-dvr #10(w337) -> (w320:errorcluster)  [unwired: 1 out]
        }
        n128 = Merge Errors(w323, w320) -> (w321:errorcluster)
      }
      event "remap": Value Change {
        n129 = event-data() -> ()  [unwired: 1 in, 1 out]
        n130 = Generate User Event(user event=w347, event data cluster=T7 {"command"="Refresh", "data"=""} ("event data")) -> ()  [unwired: 2 in, 2 out]
        n131 = in-place {
          in-place-border: w349 -> [w358]
          in-place-border: "mapping" -> [w357]
          in-place-border: [w356] -> w345
          n132 = in-place-dvr #11(w342) -> (w351:refnum<class "Modbus Slave editor node.lvclass">, w354:errorcluster)
          n133 = Unbundle By Name(w351) -> ("module configuration"=w353:refnum<class "Modbus Slave configuration.lvclass">)
          n134 = Merge Errors(w358, w354) -> (w355:errorcluster)
          n135 = call "map Modbus channels.vi"("error in"=w355, "mapping"=w357, "Modbus Slave configuration in"=w353) -> ("error out"=w356:errorcluster, "Modbus Slave configuration out"=w352:refnum<class "Modbus Slave configuration.lvclass">)  [unwired: 7 in]
          n136 = Bundle By Name(cluster=w351, "module configuration"=w352) -> (w350:refnum<class "Modbus Slave editor node.lvclass">)
          n137 = in-place-dvr #11(w350) -> (w343:errorcluster)  [unwired: 1 out]
        }
        n138 = Merge Errors(w345, w343) -> (w344:errorcluster)
      }
      event "channel": Shortcut Menu Activation? {
        n139 = event-data() -> ("MenuRef"=w369:refnum<k9>, "CtlRef"=w371:refnum<vi>, "Coords"=w370:T10)  [unwired: 1 in]
        n140 = invoke class="MCListbox (strict)" method="Point To Row Column"(reference=w371, "Point"=w370) -> (reference out=w368:refnum<vi>, error out=w367:errorcluster, "CellPosition"=w366:T11)  [unwired: 5 in, 4 out]
        n141 = Delete Menu Items(6:w373, 9:w369) -> (0:w360:errorcluster, 3:w361:refnum<k9>)  [unwired: 2 in]
        n142 = Unbundle(w366) -> ("Row"=w364:i32)  [unwired: 1 out]
        n143 = property class="MCListbox (strict)"(reference=w368, error in=w367) -> ("ItemNames"=w365:string[][])  [unwired: 2 out]
        n144 = Index Array(array=w365, index (row)=w364, index (col)=0 ("disabled index (col)")) -> (element=w362:string)
        n145 = case shown="Default" w362 {
          tunnel: w361 -> [w377 w381]
          tunnel: w360 -> [w376 w380]
          tunnel: [w375 w379] -> w359
          frame Default {
            w374 = string[] ["Add", "Edit", "Delete"] ("item names")
            n146 = Insert Menu Items(6:w376, 7:w374, 8:w374, 9:w377) -> (0:w375:errorcluster)  [unwired: 2 in, 2 out]
          }
          frame "" {
            w378 = string[] ["Add"] ("item names")
            n147 = Insert Menu Items(6:w380, 7:w378, 8:w378, 9:w381) -> (0:w379:errorcluster)  [unwired: 2 in, 2 out]
          }
        }
        n148 = event-data("Discard?"=FALSE) -> ()  [unwired: 1 in, 1 out]
      }
      event "channel": Shortcut Menu Selection (User) {
        n149 = event-data() -> ("ItemTag"=w387:string, "CtlRef"=w388:refnum<vi>, "Coords"=w389:T10)  [unwired: 1 in]
        n150 = invoke class="MCListbox (strict)" method="Point To Row Column"(reference=w388, "Point"=w389) -> ("CellPosition"=w383:T11)  [unwired: 5 in, 6 out]
        n151 = Unbundle By Name(w383) -> ("Row"=w382:i32)
        n152 = property on="channel" class="MCListbox (strict)"(error in=w385, "Value"=w382) -> (error out=w384:errorcluster)  [unwired: 1 in, 1 out]
        n153 = case shown="\"Delete\"" w387 {
          tunnel: w384 -> [w390 w392 w396 w399]
          tunnel: [w390 w391 w395 w398] -> w386
          frame Default {
          }
          frame "Add" {
            n154 = property on="hidden_Add" class="Bool (strict)"(error in=w392, "Val(Sgnl)"=TRUE ("Value (Signaling)")) -> (error out=w391:errorcluster)  [unwired: 1 in, 1 out]
          }
          frame "Edit" {
            n155 = property on="hidden_settings" class="Bool (strict)"(error in=w396, "Val(Sgnl)"=TRUE ("Value (Signaling)")) -> (error out=w395:errorcluster)  [unwired: 1 in, 1 out]
          }
          frame "Delete" {
            n156 = property on="hidden_remove" class="Bool (strict)"(error in=w399, "Val(Sgnl)"=FALSE ("Value (Signaling)")) -> (error out=w398:errorcluster)  [unwired: 1 in, 1 out]
          }
        }
      }
      event "export": Value Change {
        n157 = event-data() -> ()  [unwired: 1 in, 1 out]
        n158 = property class="Modbus Slave editor node"(reference=w406, error in=w413) -> (error out=w407:errorcluster, "Data Access:Module Configuration"=w403:refnum<class "TBM module configuration.lvclass">)  [unwired: 1 out]
        n159 = To More Specific Class(target class=refnum<class "Modbus Slave configuration.lvclass"> refnum ("tag bus configurable plugin module configuration"), reference=w403, error in=w407) -> (specific class reference=w402:refnum<class "Modbus Slave configuration.lvclass">, error out=w404:errorcluster)
        n160 = property class="Modbus Slave configuration"(reference=w402, error in=w404) -> (error out=w405:errorcluster, "data access:modbus channels"=w400:refnum<class "Modbus Module Channel.lvclass">[])  [unwired: 1 out]
        n161 = call "File Dialog"("error in"=w405, "pattern (all files)"="*.csv") -> ("selected path"=w412:path, "cancelled"=w409:bool, "error out"=w410:errorcluster)  [unwired: 10 in, 1 out]
        n162 = case shown="False" w409 {
          tunnel: w412 -> [w415 _]
          tunnel: w410 -> [w416 w418]
          tunnel: [w417 w418] -> w408
          tunnel: w400 -> [w414 _]
          frame False {
            n163 = call "export csv to kepserverex.vi"("error in"=w416, "modbus channels"=w414, "selected path"=w415) -> ("error out"=w417:errorcluster)  [unwired: 8 in]
          }
          frame True {
          }
        }
      }
    }
    n164 = case shown="No Error" w73 {
      selector: w73 -> [w84 w88]
      tunnel: [w85 w89] -> w80
      tunnel: w71 -> [w85 w89]
      tunnel: [w84 w86] -> w79
      frame No Error {
      }
      frame Error {
        n165 = call <vilib>:"Simple Error Handler.vi"("error in (no error)"=w88) -> ("error out"=w87:errorcluster)  [unwired: 4 in, 4 out]
        n166 = call <vilib>:"Clear Errors.vi"("error in (no error)"=w87) -> ("error out"=w86:errorcluster)  [unwired: 6 in]
      }
    }
  }
  n167 = Unregister For Events(event registration refnum=w35, error in=w34) -> (error out=w20:errorcluster)
  n168 = call <vilib>:"Simple Error Handler.vi"("error in (no error)"=w20) -> ()  [unwired: 4 in, 5 out]
